vi "2526 Parse Scan List.vi"(11 "MUX Input String":string="ch0:6") -> (3 "Channel Array":string[](array[string]))   [LabVIEW 2019, in "SupportVIs.lvlib"]
uses:
  SupportVIs.lvlib
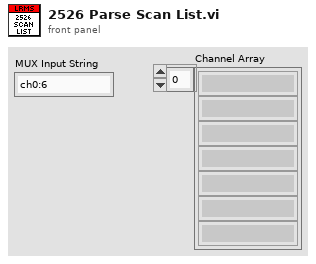
[diagram p1: front panel]
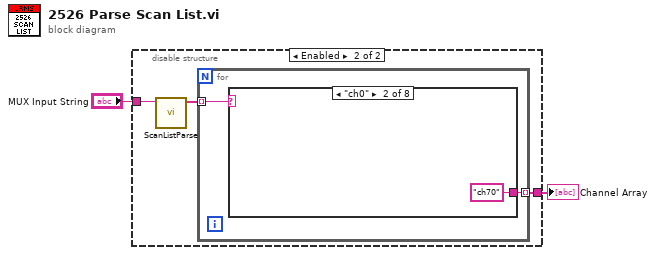
[diagram p0: block diagram]
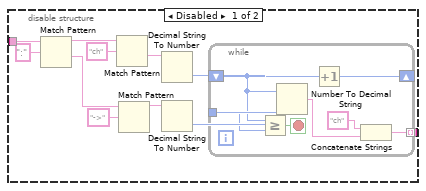
[diagram p2: hidden frame]
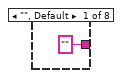
[diagram p3: hidden frame]
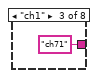
[diagram p4: hidden frame]
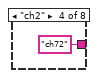
[diagram p5: hidden frame]
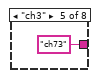
[diagram p6: hidden frame]
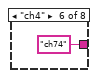
[diagram p7: hidden frame]
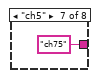
[diagram p8: hidden frame]
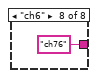
[diagram p9: hidden frame]
diagram:
  n1 = disable-structure shown="Enabled" {
    disable-tunnel: "MUX Input String" -> [w13 w23]
    disable-tunnel: [w3 w21] -> w1
    frame Disabled {
      n2 = Match Pattern(string=w13, regular expression=":" ("search string")) -> (before substring=w8:string, after substring=w11:string)  [unwired: 1 in, 2 out]
      n3 = Match Pattern(string=w8, regular expression="ch") -> (after substring=w7:string)  [unwired: 1 in, 3 out]
      n4 = Match Pattern(string=w11, regular expression="->") -> (before substring=w6:string)  [unwired: 1 in, 3 out]
      n5 = Decimal String To Number(string=w7) -> (number=w4:i32)  [unwired: 2 in, 1 out]
      n6 = Decimal String To Number(string=w6) -> (number=w5:i32)  [unwired: 2 in, 1 out]
      n7 = while {
        tunnel: w5 -> [w20]
        shift-right: [w18] -> _
        shift-left: w4 -> [w17]
        tunnel: [w14] -> w3 mode=indexing
        stop <- w19 stop-if-true
        n8 = Greater Or Equal?(x=w17, y=w20) -> (x >= y?=w19:bool)
        n9 = Number To Decimal String(number=w17) -> (decimal integer string=w15:string)  [unwired: 1 in]
        n10 = Increment(x=w17) -> (x+1=w18:i32)
        n11 = Concatenate Strings("ch" ("string"), w15) -> (w14:string)
      }
    }
    frame Enabled {
      n12 = call "ScanListParse.vi"("Input"=w23) -> ("Output"=w22:string[])  [unwired: 10 in]
      n13 = for {
        tunnel: w22 -> [w25] mode=indexing
        tunnel: [w24] -> w21 mode=indexing
        n14 = case shown="\"ch0\"" w25 {
          tunnel: ["" "ch70" "ch71" "ch72" "ch73" "ch74" "ch75" "ch76"] -> w24
          frame "", Default {
          }
          frame "ch0" {
          }
          frame "ch1" {
          }
          frame "ch2" {
          }
          frame "ch3" {
          }
          frame "ch4" {
          }
          frame "ch5" {
          }
          frame "ch6" {
          }
        }
      }
    }
  }
  "Channel Array" <- w1
